vi "SubVI_formula.vi"(9 "b":dbl, 10 "a":dbl, 11 "x":dbl) -> (3 "y":dbl)   [LabVIEW 2018]
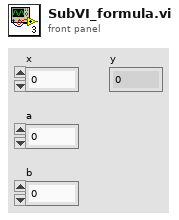
[diagram p1: front panel]
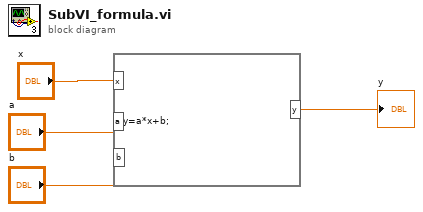
[diagram p0: block diagram]
diagram:
  n1 = formula code="y=a*x+b;"("x"="x", "a"="a", "b"="b") -> ("y"=→"y":dbl)
